vi "Execute.vi"(8 "error in (no error)":errorcluster, 11 "Stop Low Pressure Wax in":refnum<class "Stop Low Pressure Wax.lvclass">) -> (0 "error out":errorcluster, 3 "Stop Low Pressure Wax out":refnum<class "Stop Low Pressure Wax.lvclass">)   [LabVIEW 2019, in "Stop Low Pressure Wax.lvclass"]
uses:
  <vilib>/gpm_packages/@cs/Car-wash/Source/Process Steps/Stop Low Pressure Wax/Stop Low Pressure Wax.lvclass
  C:/Program Files/National Instruments/LabVIEW 2019/vi.lib/gpm_packages/@cs/mva-core/Source/IModel/IModel/IModel.lvclass
  C:/Program Files/National Instruments/LabVIEW 2019/vi.lib/ActorFramework/Actor/Actor.lvclass
  <vilib>/gpm_packages/@cs/Car-wash/Source/Process Steps/Stop Low Pressure Wax/Stop Low Pressure Wax.lvclass/Stop Low Pressure Wax.ctl
  <vilib>/gpm_packages/@cs/mva-core/Source/IObserver/IObserver/IObserver.lvclass/IObserver.ctl
  <vilib>/gpm_packages/@cs/mva-core/Source/IModel/IModel/IModel.lvclass/IModel.ctl
  <vilib>/gpm_packages/@cs/mva-core/Source/IMediator/PublishRequest/PublishRequest.lvclass/PublishRequest.ctl
  <vilib>/gpm_packages/@cs/mva-core/Source/IMediator/IMediator Messages/Publish Msg/Publish Msg.lvclass/Publish Msg.ctl
  <vilib>/gpm_packages/@cs/actor-framework-messages/Source/RoundTripMessage/RoundTripMessage.lvclass/RoundTripMessage.ctl
  <vilib>/ActorFramework/Message Enqueuer/Message Enqueuer.lvclass/Message Enqueuer.ctl
  <vilib>/ActorFramework/Actor/Actor.lvclass/Actor.ctl
  <vilib>/gpm_packages/@cs/mva-core/Source/IMediator/IMediator Messages/Publish Msg/Send Pre-Addressed Publish.vi
  <vilib>/gpm_packages/@cs/mva-core/Source/IObserver/IObserver/Read Unique ID.vi
  <vilib>/gpm_packages/@cs/mva-core/Source/IMediator/PublishRequest/Pack Publish Request.vi
  <vilib>/ActorFramework/Message Enqueuer/Init from Existing Queue.vi
  <vilib>/ActorFramework/Message Enqueuer/Enqueue.vi
  <vilib>/gpm_packages/@cs/actor-framework-messages/Source/RoundTripMessage/Return Round-Trip Message.vi
  <vilib>/gpm_packages/@cs/mva-core/Source/IModel/IModel/IModel.lvclass
  C:/Program Files/National Instruments/LabVIEW 2019/vi.lib/gpm_packages/@cs/mva-core/Source/IObserver/IObserver/IObserver.lvclass
  <vilib>/gpm_packages/@cs/mva-core/Source/IMediator/IMediator Messages/Publish Msg/Publish Msg.lvclass
  C:/Program Files/National Instruments/LabVIEW 2019/vi.lib/gpm_packages/@cs/actor-framework-messages/Source/RoundTripMessage/RoundTripMessage.lvclass
  <vilib>/gpm_packages/@cs/actor-framework-messages/Source/RoundTripMessage/RoundTripMessage.lvclass
  C:/Program Files/National Instruments/LabVIEW 2019/vi.lib/ActorFramework/Message/Message.lvclass
  <vilib>/ActorFramework/Stop Msg/Stop Msg.lvclass
  <vilib>/Utility/error.llb/Error Cluster From Error Code.vi
  <vilib>/ActorFramework/Message Priority Queue/Priority Enqueue.vi
  <vilib>/gpm_packages/@cs/mva-core/Source/IMediator/PublishRequest/PublishRequest.lvclass
  <vilib>/ActorFramework/Message Enqueuer/Message Enqueuer.lvclass
  <vilib>/ActorFramework/Actor/Actor.lvclass
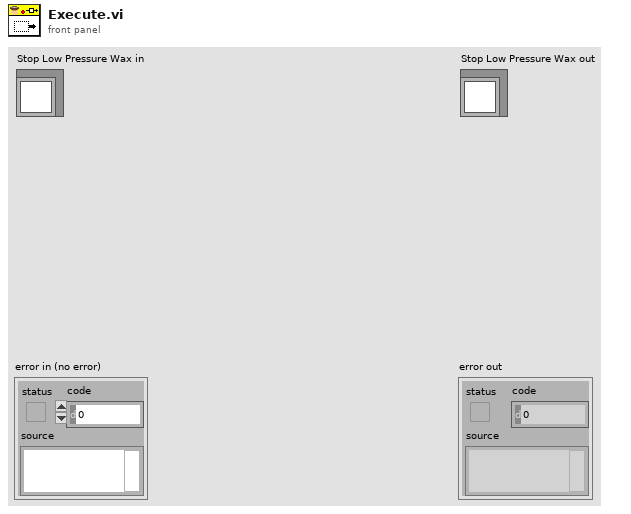
[diagram p1: front panel]
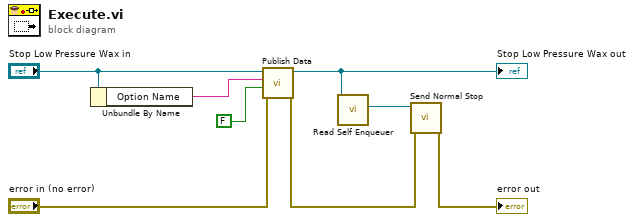
[diagram p0: block diagram]
diagram:
  n1 = Unbundle By Name("Stop Low Pressure Wax in") -> ("Option Name"=w7:string)
  n2 = call <vilib>:"Publish Data.vi"("error in (no error)"="error in (no error)", "Data to Publish"=FALSE, "Datum Name"=w7, "IModel in"="Stop Low Pressure Wax in") -> ("error out"=w2:errorcluster, "IModel out"=w4:refnum<class "Stop Low Pressure Wax.lvclass">)  [unwired: 6 in]
  "Stop Low Pressure Wax out" <- w4
  n3 = call <vilib>:"Read Self Enqueuer.vi"("Actor"=w4) -> ("Self Enqueuer"=w8:refnum<class "Message Enqueuer.lvclass">)  [unwired: 10 in]
  n4 = call <vilib>:"Send Normal Stop.vi"("error in (no error)"=w2, "Message Enqueuer"=w8) -> ("error out"=→"error out":errorcluster)  [unwired: 9 in]
